vi "Setup DCPower Voltage.vi"(7 "Channel Groups?":bool, 8 "error in":errorcluster, 9 "Parameters":T1={"Supply"=0.0, "Limit"=0.0, "Aperture Time"=0.0, "Settling Time"=0.0, "Sense"=1008, "Transient Response"=1041} {"Transient Response" items=["Slow"=1041, "Normal"=1038, "Fast"=1039, "Custom"=1042]; "Sense" items=["Local"=1008, "Remote"=1009]}, 10 "Channel List":string, 11 "DCPower Handle In":refnum<k15>) -> (0 "error out":errorcluster, 3 "DCPower Handle Out":refnum<k15>)   [LabVIEW 2021, in "PMIC Common.lvlib"]
uses:
  PMIC Common.lvlib
  DCPower Parameters.ctl
  <instrlib>/niDCPower/nidcpower.llb/niDCPower Output Function.ctl
  <instrlib>/niDCPower/nidcpower.llb/niDCPower Source Mode.ctl
  <instrlib>/niDCPower/nidcpower.llb/niDCPower Wait For Event - Event.ctl
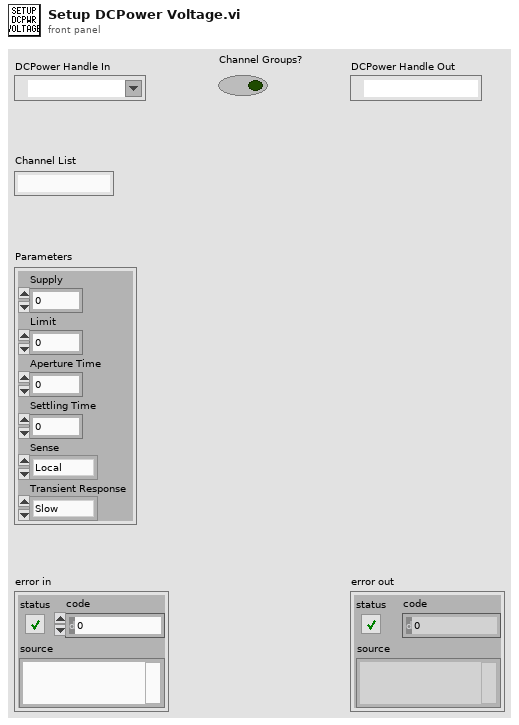
[diagram p1: front panel]
types:
  T1 = typedef "PMIC Common.lvlib/DCPower Parameters.ctl" = cluster{"Supply":dbl, "Limit":dbl, "Aperture Time":dbl, "Settling Time":dbl, "Sense":i32, "Transient Response":i32}
  T2 = typedef "niDCPower Source Mode.ctl" = i32
  T3 = typedef "niDCPower Output Function.ctl" = i32
  T4 = typedef "niDCPower Wait For Event - Event.ctl" = i32
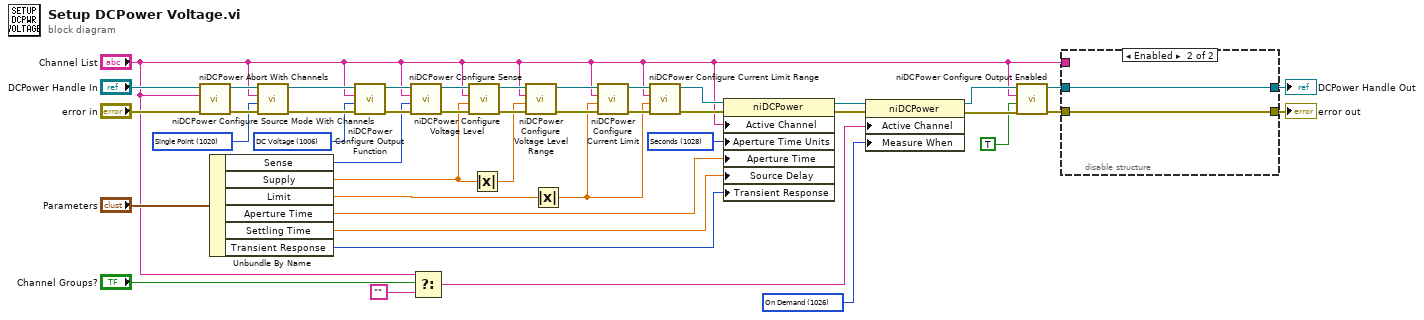
[diagram p0: block diagram]
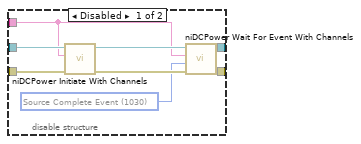
[diagram p2: hidden frame]
diagram:
  w16 = 1026 items=["Automatically after Source Complete"=1025, "On Demand"=1026, "On Measure Trigger"=1027] ("Measurement:Advanced:Measure When")
  w31 = T2 1020 items=["Single Point"=1020, "Sequence"=1021] ("source mode")
  w35 = 1028 items=["Seconds"=1028, "Power Line Cycles"=1029] ("Measurement:Aperture Time Units")
  w3 = T3 1006 items=["DC Voltage"=1006, "DC Current"=1007, "Pulse Voltage"=1049, "Pulse Current"=1050] ("output function")
  n1 = call <instrlib>:"niDCPower Abort With Channels.vi"("error in (no error)"="error in", "channel name"="Channel List", "instrument handle"="DCPower Handle In") -> ("error out"=w33:errorcluster, "instrument handle out"=w44:refnum<k15>)  [unwired: 7 in]
  n2 = Unbundle By Name("Parameters") -> ("Sense"=w9:i32, "Supply"=w8:dbl, "Limit"=w7:dbl, "Aperture Time"=w6:dbl, "Settling Time"=w5:dbl, "Transient Response"=w4:i32)
  n3 = call <instrlib>:"niDCPower Configure Source Mode With Channels.vi"("error in (no error)"=w33, "source mode"=w31, "channel name"="Channel List", "instrument handle"=w44) -> ("error out"=w32:errorcluster, "instrument handle out"=w34:refnum<k15>)  [unwired: 6 in]
  n4 = call <instrlib>:"niDCPower Configure Output Function.vi"("error in (no error)"=w32, "output function"=w3, "channel name"="Channel List", "instrument handle"=w34) -> ("error out"=w27:errorcluster, "instrument handle out"=w26:refnum<k15>)  [unwired: 6 in]
  n5 = call <instrlib>:"niDCPower Configure Sense.vi"("error in (no error)"=w27, "sense"=w9, "channel name"="Channel List", "instrument handle"=w26) -> ("error out"=w24:errorcluster, "instrument handle out"=w25:refnum<k15>)  [unwired: 6 in]
  n6 = Select(t="Channel List", s="Channel Groups?", f="") -> (s? t:f=w17:string)
  n7 = call <instrlib>:"niDCPower Configure Voltage Level.vi"("error in (no error)"=w24, "voltage level"=w8, "channel name"="Channel List", "instrument handle"=w25) -> ("error out"=w43:errorcluster, "instrument handle out"=w42:refnum<k15>)  [unwired: 6 in]
  n8 = Absolute Value(x=w8) -> (abs(x)=w23:dbl)
  n9 = call <instrlib>:"niDCPower Configure Voltage Level Range.vi"("error in (no error)"=w43, "voltage level range"=w23, "channel name"="Channel List", "instrument handle"=w42) -> ("error out"=w39:errorcluster, "instrument handle out"=w38:refnum<k15>)  [unwired: 6 in]
  n10 = Absolute Value(x=w7) -> (abs(x)=w28:dbl)
  n11 = call <instrlib>:"niDCPower Configure Current Limit.vi"("error in (no error)"=w39, "current limit"=w28, "channel name"="Channel List", "instrument handle"=w38) -> ("error out"=w41:errorcluster, "instrument handle out"=w40:refnum<k15>)  [unwired: 6 in]
  n12 = call <instrlib>:"niDCPower Configure Current Limit Range.vi"("error in (no error)"=w41, "current limit range"=w28, "channel name"="Channel List", "instrument handle"=w40) -> ("error out"=w36:errorcluster, "instrument handle out"=w37:refnum<k15>)  [unwired: 6 in]
  n13 = property class="niDCPower"(reference=w37, error in=w36, "Active Channel"="Channel List", "Aperture Time Units"=w35, "Aperture Time"=w6, "Source Delay"=w5, "Transient Response"=w4) -> (reference out=w20:refnum<k15>, error out=w22:errorcluster)
  n14 = property class="niDCPower"(reference=w20, error in=w22, "Active Channel"=w17, "Measure When"=w16) -> (reference out=w21:refnum<k15>, error out=w19:errorcluster)
  n15 = call <instrlib>:"niDCPower Configure Output Enabled.vi"("error in (no error)"=w19, "output enabled"=TRUE, "channel name"="Channel List", "instrument handle"=w21) -> ("error out"=w30:errorcluster, "instrument handle out"=w29:refnum<k15>)  [unwired: 6 in]
  n16 = disable-structure shown="Enabled" {
    disable-tunnel: w30 -> [w49 w53]
    disable-tunnel: w29 -> [w48 w54]
    disable-tunnel: [w47 w53] -> w12
    disable-tunnel: [w46 w54] -> w11
    disable-tunnel: "Channel List" -> [w45 _]
    frame Disabled {
      w50 = T4 1030 items=["Source Complete Event"=1030, "Measure Complete Event"=1031, "Sequence Iteration Complete Event"=1032, "Sequence Engine Done Event"=1033, "Pulse Complete Event"=1051, "Ready For Pulse Trigger Event"=1052] ("event")
      n17 = call <instrlib>:"niDCPower Initiate With Channels.vi"("error in (no error)"=w49, "channel name"=w45, "instrument handle"=w48) -> ("error out"=w51:errorcluster, "instrument handle out"=w52:refnum<k15>)  [unwired: 7 in]
      n18 = call <instrlib>:"niDCPower Wait For Event With Channels.vi"("error in (no error)"=w51, "event"=w50, "channel name"=w45, "instrument handle"=w52) -> ("error out"=w47:errorcluster, "instrument handle out"=w46:refnum<k15>)  [unwired: 6 in]
    }
    frame Enabled {
    }
  }
  "error out" <- w12
  "DCPower Handle Out" <- w11
